vi "Cluster.vi"() -> ()   [LabVIEW 2017]
panel:
  out "Cluster":T1
  in  "Student Data":T2
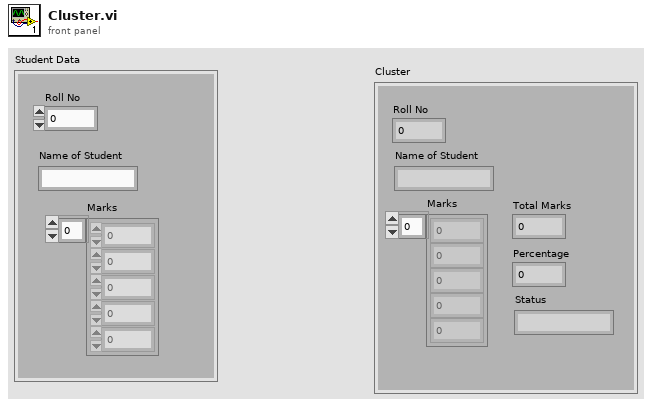
[diagram p1: front panel]
types:
  T1 = cluster{"Roll No":dbl, "Name of Student":string, "Marks":dbl[], "Total Marks":dbl, "Percentage":dbl, "Status":string}
  T2 = cluster{"Roll No":dbl, "Name of Student":string, "Marks":dbl[]}
  T3 = cluster{"Roll No":dbl, "Name of Student":string, "Marks":dbl[], "Numeric":dbl, dbl, string}
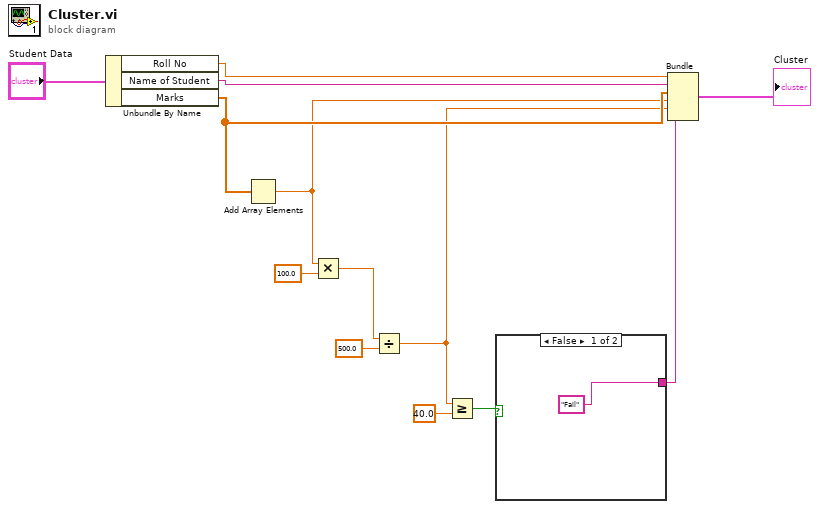
[diagram p0: block diagram]
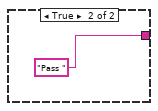
[diagram p2: hidden frame]
diagram:
  n1 = Unbundle By Name("Student Data") -> ("Roll No"=w6:dbl, "Name of Student"=w5:string, "Marks"=w4:dbl[])
  n2 = Add Array Elements(numeric array=w4) -> (sum=w3:dbl)
  n3 = Multiply(x=w3, y=100.0) -> (x*y=w11:dbl)
  n4 = Divide(x=w11, y=500.0) -> (x/y=w2:dbl)
  n5 = Greater Or Equal?(x=w2, y=40.0) -> (x >= y?=w8:bool)
  n6 = case shown="False" w8 {
    tunnel: ["Fail" "Pass "] -> w1
    frame False {
    }
    frame True {
    }
  }
  n7 = Bundle("Roll No"=w6, "Name of Student"=w5, "Marks"=w4, "Numeric"=w3, w2, w1) -> (→"Cluster":T3)  [unwired: 1 in]
